vi "Asylum_GetGroupLabels.vi"(8 "error in (no error)":errorcluster, 9 "textWave":string, 10 "groupName":string, 11 "Application":refnum<k7>) -> (0 "error out":errorcluster, 2 "Group Labels":string, 3 "Application":refnum<k7>)   [LabVIEW 2019]
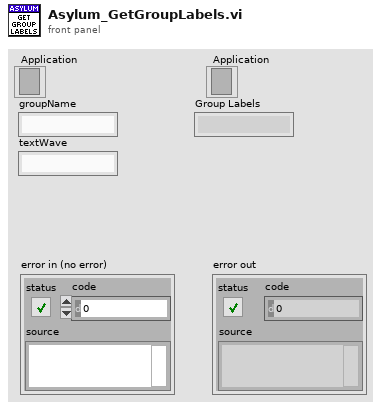
[diagram p1: front panel]
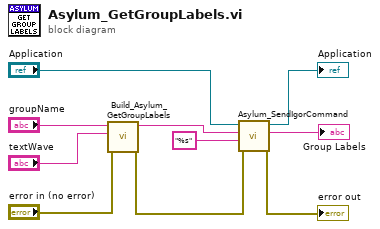
[diagram p0: block diagram]
diagram:
  n1 = call "Build_Asylum_GetGroupLabels.vi"("error in (no error)"="error in (no error)", "textWave"="textWave", "groupName"="groupName") -> ("error out"=w10:errorcluster, "Command"=w8:string)  [unwired: 7 in]
  n2 = call "Asylum_SendIgorCommand.vi"("error in (no error)"=w10, "Format"="%s", "command"=w8, "Application In"="Application") -> ("error out"=→"error out":errorcluster, "results"=→"Group Labels":string, "Application Out"=→"Application":refnum<k7>)  [unwired: 4 in, 1 out]
